vi "test udp++.vi"() -> ()   [LabVIEW 2017]
uses:
  16e1070c-7dc9-4f03-9a7c-c4bc31601776.vi
  dd86c118-00dc-4621-9a13-23dbe0247810.vi
  <vilib>/Utility/High Resolution Relative Seconds.vi
  16e1070c-7dc9-4f03-9a7c-c4bc31601776.vi/c01658a1-883f-489e-b376-c551e55a1c83.vi
  16e1070c-7dc9-4f03-9a7c-c4bc31601776.vi/6e636c19-7630-4ea6-b6f9-ce8a82b84073.vi
  16e1070c-7dc9-4f03-9a7c-c4bc31601776.vi/568dc0bf-3eb4-4251-8007-07b1324b2ce9.vi
  dd86c118-00dc-4621-9a13-23dbe0247810.vi/f576cfcf-0274-437d-9d31-e81457e56e77.vi
  SplitUDPPacks.vi
panel:
  in  "stop":bool
  out "sumcheck 2":dbl[](array[numeric])
  out "sumcheck":dbl
  out "# Count":i64[](array[numeric])
  out "time diff(s)":dbl
  in  "Numeric":i32=500
  out "Array":sgl[](array[numeric])
  out "接收控制指令":sgl[](array[numeric])
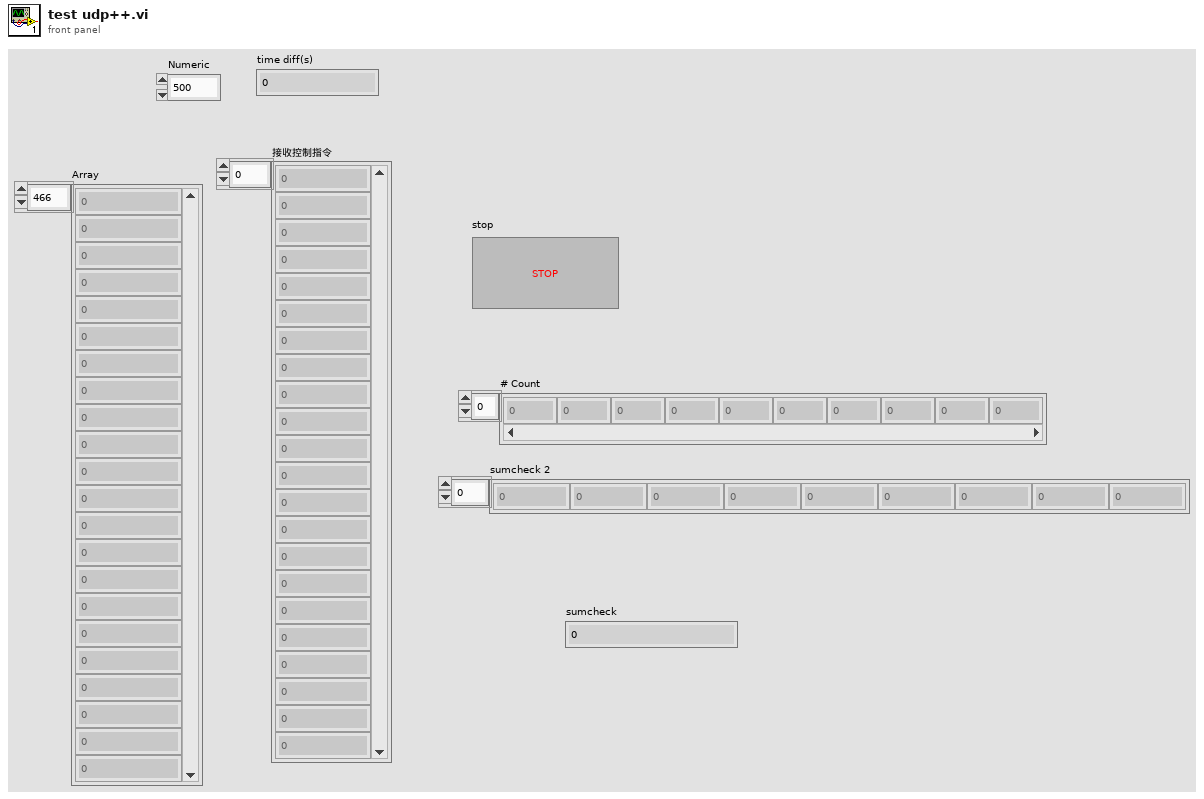
[diagram p1: front panel]
types:
  T1 = cluster{"本地IP":string, "本地端口":u16, "远程IP":string, "远程端口":u16}
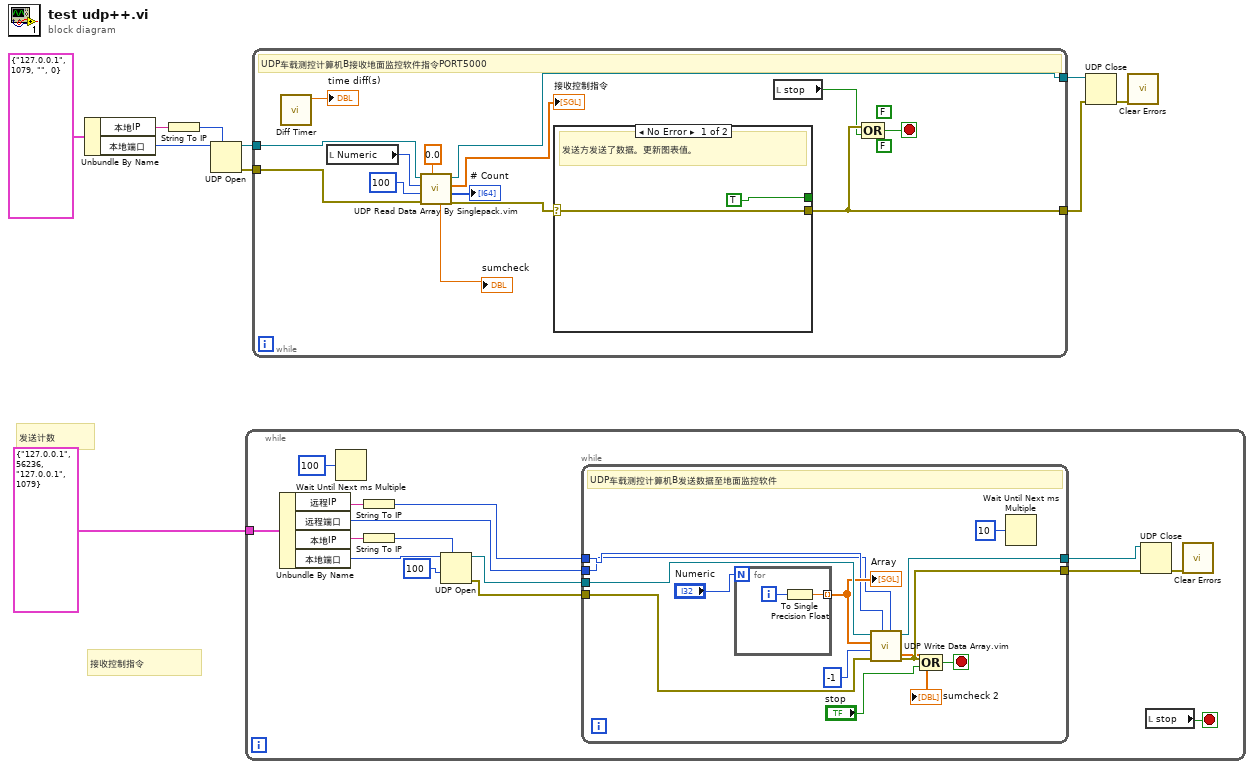
[diagram p0: block diagram]
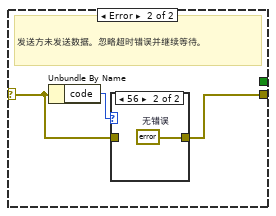
[diagram p2: hidden frame]
diagram:
  # "发送计数"
  # "接收控制指令"
  n1 = Unbundle By Name(T1 {"本地IP"="127.0.0.1", "本地端口"=1079, "远程IP"="", "远程端口"=0} ("UDP配置")) -> ("本地IP"=w3:string, "本地端口"=w2:u16)
  n2 = String To IP(1:w3) -> (0:w10:u32)
  n3 = UDP Open(7:w10, 11:w2) -> (port=w9:refnum<k16>, 0:w8:errorcluster)  [unwired: 3 in, 1 out]
  n4 = while {
    tunnel: T1 {"本地IP"="127.0.0.1", "本地端口"=56236, "远程IP"="127.0.0.1", "远程端口"=1079} ("UDP配置") -> [w16]
    stop <- w11 stop-if-true
    n5 = Unbundle By Name(w16) -> ("远程IP"=w13:string, "远程端口"=w12:u16, "本地IP"=w14:string, "本地端口"=w15:u16)
    n6 = Wait Until Next ms Multiple(millisecond multiple=u32 100 ("毫秒倍数")) -> ()  [unwired: 1 out]
    n7 = String To IP(1:w13) -> (0:w21:u32)
    n8 = String To IP(1:w14) -> (0:w23:u32)
    n9 = UDP Open(7:w23, 9:100 ("超时毫秒(25000)"), 11:w15) -> (port=w25:refnum<k16>, 0:w24:errorcluster)  [unwired: 2 in, 1 out]
    n10 = while {
      tunnel: [w35] -> w19
      tunnel: w25 -> [w38]
      tunnel: w24 -> [w36]
      tunnel: [w37] -> w18
      tunnel: w12 -> [w30]
      tunnel: w21 -> [w31]
      stop <- w34 stop-if-true
      # "UDP车载测控计算机B发送数据至地面监控软件"
      n11 = for {
        N: "Numeric" -> [_]
        tunnel: [w39] -> w32 mode=indexing
        i -> [w40]
        n12 = To Single Precision Float(number=w40) -> (single precision float=w39:sgl)
      }
      "Array" <- w32
      n13 = call "UDP Write Data Array.vim"("port or service name"=w30, "address"=w31, "error in (no error)"=w36, "超时毫秒(25000)"=-1, "Data"=w32, "UDP Network Connection in"=w38) -> ("error out"=w35:errorcluster, "UDP Network Connection out"=w37:refnum<k16>, "checksum"=→"sumcheck 2":dbl[])  [unwired: 3 in]
      n14 = Compound Arithmetic op=OR ("复合运算")(w35, "stop") -> (w34:bool)
      n15 = Wait Until Next ms Multiple(millisecond multiple=u32 10 ("毫秒倍数")) -> ()  [unwired: 1 out]
    }
    n16 = UDP Close(connection ID=w18, 8:w19) -> (error out=w17:errorcluster)  [unwired: 1 out]
    n17 = local read "stop"() -> (w11:bool)
    n18 = call <vilib>:"Clear Errors.vi"("error in (no error)"=w17) -> ()  [unwired: 5 in, 2 out]
  }
  n19 = while {
    tunnel: w9 -> [w54]
    tunnel: [w52] -> w6
    tunnel: w8 -> [w53]
    tunnel: [w51] -> w7
    stop <- w50 stop-if-true
    (unwired) FALSE ("reset value")
    (unwired) FALSE ("reset")
    # "UDP车载测控计算机B接收地面监控软件指令PORT5000"
    n20 = call "Diff Timer.vi"() -> ("time diff(s)"=→"time diff(s)":dbl)  [unwired: 10 in, 1 out]
    n21 = local read "Numeric"() -> (w46:i32)
    n22 = call "UDP Read Data Array By Singlepack.vim"("Data Type(dbl)"=sgl 0.0, "error in (no error)"=w53, "超时毫秒(25000)"=100 ("timeout ms (25000)"), "total size"=w46, "UDP Network Connection in"=w54) -> ("error out"=w48:errorcluster, "# Count"=→"# Count":i64[], "Array"=→"接收控制指令":sgl[], "UDP Network Connection out"=w52:refnum<k16>, "checksum"=→"sumcheck":dbl)  [unwired: 2 in]
    n23 = case shown="No Error" w48 {
      selector: w48 -> [w56 w58]
      tunnel: [w56 w57] -> w51
      tunnel: [TRUE ("wifi_KongZ") _] -> _
      frame No Error {
        # "发送方发送了数据。更新图表值。"
      }
      frame Error {
        # "发送方未发送数据。忽略超时错误并继续等待。"
        n24 = Unbundle By Name(w58) -> ("code"=w59:i32)
        n25 = case shown="56" w59 {
          tunnel: w58 -> [w60 _]
          tunnel: [w60 w61] -> w57
          frame Default {
          }
          frame 56 {
            w61 = errorcluster {"status"=FALSE, "code"=0, "source"=""}  # 无错误
          }
        }
      }
    }
    n26 = local read "stop"() -> (w41:bool)
    n27 = Compound Arithmetic op=OR ("复合运算")(w51, w41) -> (w50:bool)
  }
  n28 = UDP Close(connection ID=w6, 8:w7) -> (error out=w5:errorcluster)  [unwired: 1 out]
  n29 = call <vilib>:"Clear Errors.vi"("error in (no error)"=w5) -> ()  [unwired: 5 in, 2 out]
